vi "DAQ Engine.vi"(8 "Error In":errorcluster, 10 "Output \nIndicator":T2=[FALSE, FALSE] caption="Z     Y     X", 11 "DAQ Action":T3) -> (0 "Error Out":errorcluster, 2 "Reset ?":bool, 3 "L       E \nIndicator":T1 caption="L      E")   [LabVIEW 2023]
doc: "VI for realizing DAQ action engine"
uses:
  controls/enum defining DAQ actions.ctl
  controls/Boolean output indicator.ctl
  controls/Boolean L E indictaor.ctl
  <vilib>/DAQmx/read.llb/DAQmx Read (Digital 1D Bool 1Chan 1Samp).vi
  <vilib>/DAQmx/create/channels.llb/DAQmx Create Channel (DI-Digital Input).vi
  <vilib>/DAQmx/miscellaneous.llb/DAQmx Fill In Error Info.vi
  <vilib>/DAQmx/create/channels.llb/DAQmx Create Channel (DO-Digital Output).vi
  <vilib>/DAQmx/write.llb/DAQmx Write (Digital 1D Bool 1Chan 1Samp).vi
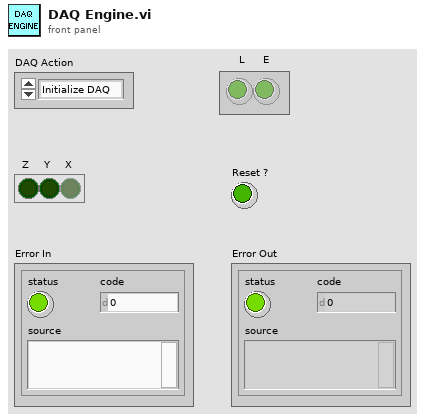
[diagram p1: front panel]
types:
  T1 = typedef "Boolean L E indictaor.ctl" = bool[]
  T2 = typedef "Boolean output indicator.ctl" = bool[]
  T3 = typedef "enum defining DAQ actions.ctl" = enum16{"Initialize DAQ", "Read L and  E  Commands", "Read R Command", "Write Outputs X, Y, and Z", "Release DAQ"}
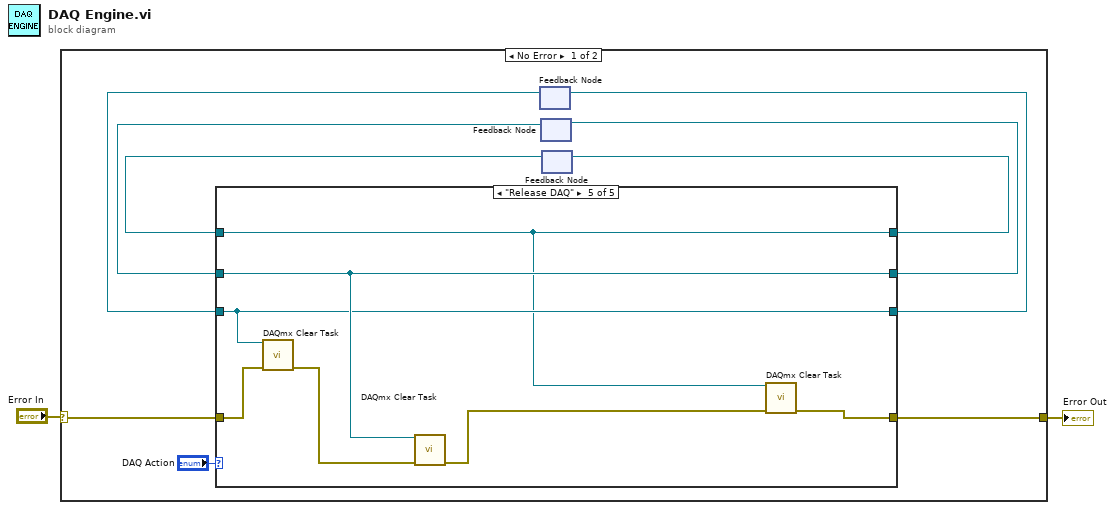
[diagram p0: block diagram]
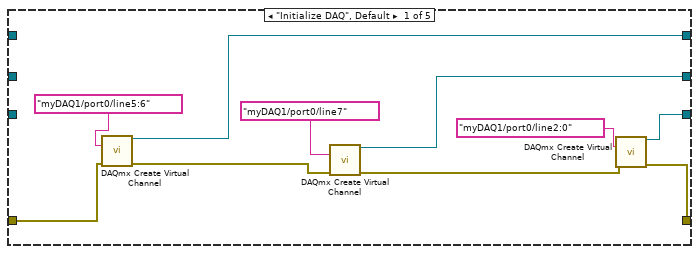
[diagram p2: hidden frame]
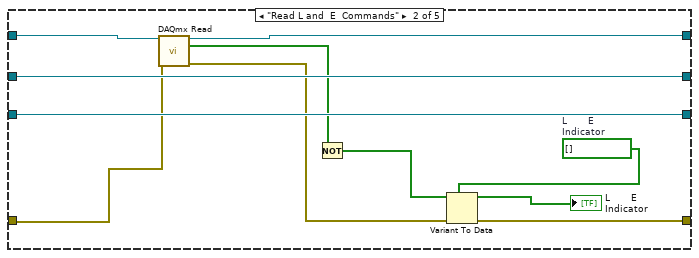
[diagram p3: hidden frame]
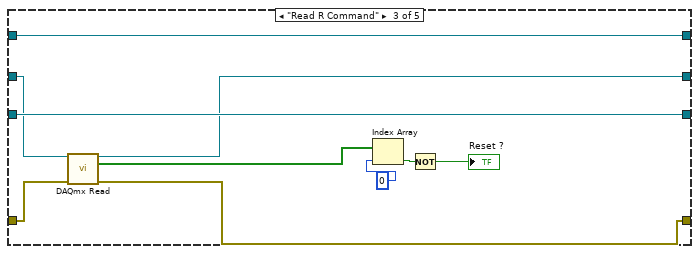
[diagram p4: hidden frame]
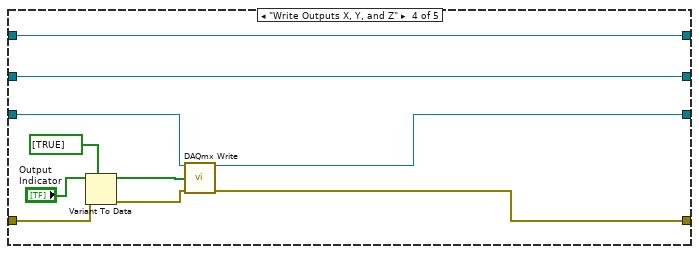
[diagram p5: hidden frame]
diagram:
  n1 = case shown="No Error" "Error In" {
    selector: "Error In" -> [w7 w60]
    tunnel: [w6 w60] -> w1
    frame No Error {
      n2 = feedback #1() -> (w4:refnum<k21>)  [unwired: 1 in]
      n3 = feedback #2() -> (w9:refnum<k21>)  [unwired: 1 in]
      n4 = feedback #3() -> (w8:refnum<k21>)  [unwired: 1 in]
      n5 = case shown="\"Release DAQ\"" "DAQ Action" {
        tunnel: [w20 w32 w39 w52 w57] -> w10
        tunnel: w9 -> [_ w32 w40 w52 w57]
        tunnel: w8 -> [_ w27 w41 w48 w53]
        tunnel: w7 -> [w19 w25 w35 w51 w56]
        tunnel: [w17 w30 w34 w49 w58] -> w6
        tunnel: [w16 w31 w42 w50 w54] -> w5
        tunnel: w4 -> [_ w31 w42 w47 w54]
        tunnel: [w15 w26 w41 w48 w53] -> w3
        frame "Initialize DAQ", Default {
          n6 = call-poly <vilib>:"DAQmx Create Virtual Channel.vi"("lines"=tag "myDAQ1/port0/line5:6", "error in"=w19) -> ("task out"=w15:refnum<k21>, "error out"=w21:errorcluster)  [unwired: 12 in]
          n7 = call-poly <vilib>:"DAQmx Create Virtual Channel.vi"("lines"=tag "myDAQ1/port0/line7", "error in"=w21) -> ("task out"=w20:refnum<k21>, "error out"=w18:errorcluster)  [unwired: 12 in]
          n8 = call-poly <vilib>:"DAQmx Create Virtual Channel.vi"("lines"=tag "myDAQ1/port0/line2:0", "error in"=w18) -> ("task out"=w16:refnum<k21>, "error out"=w17:errorcluster)  [unwired: 12 in]
        }
        frame "Read L and  E  Commands" {
          w29 = T1 []  # L       E  Indicator
          n9 = call-poly <vilib>:"DAQmx Read.vi"("task/channels in"=w27, "error in"=w25) -> ("task out"=w26:refnum<k21>, "data"=w23:bool[], "error out"=w24:errorcluster)  [unwired: 11 in]
          n10 = Not(x=w23) -> (.not. x?=w22:bool[])
          n11 = Variant To Data(error in=w24, type=w29, Variant=w22) -> (data=→"L       E \nIndicator":T1, error out=w30:errorcluster)
        }
        frame "Read R Command" {
          n12 = call-poly <vilib>:"DAQmx Read.vi"("task/channels in"=w40, "error in"=w35) -> ("task out"=w39:refnum<k21>, "data"=w38:bool[], "error out"=w34:errorcluster)  [unwired: 11 in]
          n13 = Index Array(array=w38, index=0) -> (element=w37:bool)
          n14 = Not(x=w37) -> (.not. x?=→"Reset ?":bool)
        }
        frame "Write Outputs X, Y, and Z" {
          n15 = Variant To Data(error in=w51, type=bool[] [TRUE], Variant="Output \nIndicator") -> (data=w43:bool[], error out=w44:errorcluster)
          n16 = call-poly <vilib>:"DAQmx Write.vi"("task/channels in"=w47, "data"=w43, "error in"=w44) -> ("task out"=w50:refnum<k21>, "error out"=w49:errorcluster)  [unwired: 10 in, 1 out]
        }
        frame "Release DAQ" {
          n17 = call <vilib>:"DAQmx Clear Task.vi"("task in"=w54, "error in"=w56) -> ("error out"=w55:errorcluster)  [unwired: 13 in]
          n18 = call <vilib>:"DAQmx Clear Task.vi"("task in"=w57, "error in"=w55) -> ("error out"=w59:errorcluster)  [unwired: 13 in]
          n19 = call <vilib>:"DAQmx Clear Task.vi"("task in"=w53, "error in"=w59) -> ("error out"=w58:errorcluster)  [unwired: 13 in]
        }
      }
      n20 = feedback-in #1(w5) -> ()
      n21 = feedback-in #2(w10) -> ()
      n22 = feedback-in #3(w3) -> ()
    }
    frame Error {
    }
  }
  "Error Out" <- w1
